vi "Retrieve Full Scale.vi"(8 "error in":errorcluster, 10 "Model Data":string, 11 "Alicat Device in":refnum<class "Alicat Device.lvclass">) -> (0 "error out":errorcluster, 1 "Type":string, 2 "Full Scale":sgl, 3 "Alicat Device out":refnum<class "Alicat Device.lvclass">, 4 "ModelOut":string)   [LabVIEW 2014, in "Alicat Lib.lvlib" / "Alicat Device.lvclass"]
doc: "The full scale of the device defines the input command for the setpoint (if the device is a controller). The setpoint command will use the full scale (FS) such that \n\nVal = SP*64000/FS"
uses:
  Alicat Device.lvclass
  Configurable Device/Configurable Device.lvclass/Configurable Device.ctl
  Alicat Device.lvclass/Alicat Device.ctl
  Configurable Device/Accessors/Write Model.vi
  Configurable Device/Accessors/Write SN.vi
  <vilib>/NI/Tools/String/Tools_String.lvlib
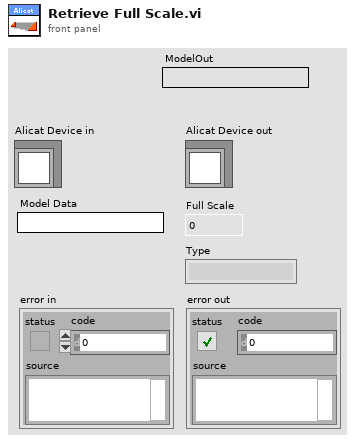
[diagram p1: front panel]
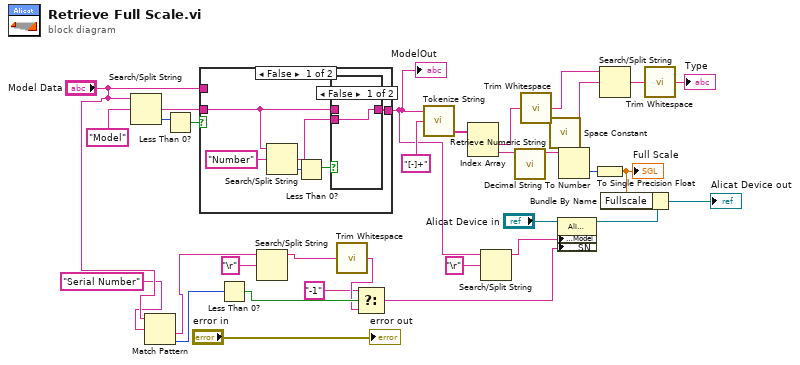
[diagram p0: block diagram]
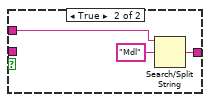
[diagram p3: hidden frame]
diagram:
  n1 = Search/Split String(string="Model Data", search string/char (-)="Model") -> (match + rest of string=w16:string, offset of match=w18:i32)  [unwired: 1 in, 1 out]
  n2 = Match Pattern(string="Model Data", regular expression="Serial Number" ("search string/char (-)")) -> (after substring=w10:string, offset past match=w9:i32)  [unwired: 1 in, 2 out]
  n3 = Less Than 0?(x=w18) -> (x < 0?=w17:bool)
  n4 = case shown="False" w17 {
    tunnel: "Model Data" -> [_ w43]
    tunnel: w16 -> [w35 _]
    tunnel: [w34 w41] -> w2
    frame False {
      n5 = Search/Split String(string=w35, search string/char (-)="Number") -> (match + rest of string=w33:string, offset of match=w37:i32)  [unwired: 1 in, 1 out]
      n6 = Less Than 0?(x=w37) -> (x < 0?=w36:bool)
      n7 = case shown="False" w36 {
        tunnel: w35 -> [_ w40]
        tunnel: [w39 w40] -> w34
        tunnel: w33 -> [w39 _]
        frame False {
        }
        frame True {
        }
      }
    }
    frame True {
      n8 = Search/Split String(string=w43, search string/char (-)="Mdl") -> (match + rest of string=w41:string)  [unwired: 1 in, 2 out]
    }
  }
  "ModelOut" <- w2
  n9 = Less Than 0?(x=w9) -> (x < 0?=w13:bool)
  n10 = Search/Split String(string=w10, search string/char (-)="\r") -> (substring before match=w7:string)  [unwired: 1 in, 2 out]
  n11 = call <vilib>:"Trim Whitespace.vi"("string"=w7) -> ("trimmed string"=w6:string)  [unwired: 1 in]
  n12 = Select(t="-1", s=w13, f=w6) -> (s? t:f=w4:string)
  n13 = call <vilib>:"Tokenize String.vi"("delimiter ([\\s\\t\\n\\r]+)"="[-]+" ("delimiter ([\\s\\t\\n\\r]+)"), "input string"=w2) -> ("token array"=w31:string[])  [unwired: 2 in, 1 out]
  n14 = Index Array(array=w31) -> (element #1=w27:string, element #2=w28:string)  [unwired: 2 in]
  n15 = Search/Split String(string=w2, search string/char (-)="\r") -> (substring before match=w1:string)  [unwired: 1 in, 2 out]
  n16 = call "Retrieve Numeric String.vi"("String in"=w28) -> ("Numeric String"=w30:string)  [unwired: 10 in]
  n17 = call <vilib>:"Trim Whitespace.vi"("string"=w27) -> ("trimmed string"=w26:string)  [unwired: 1 in]
  n18 = call <vilib>:"Space Constant.vi"() -> ("String"=w25:string)
  n19 = property class="Alicat Device"(reference="Alicat Device in", "Accessors:Model"=w1, "Accessors:SN"=w4) -> (reference out=w14:refnum<class "Alicat Device.lvclass">)  [unwired: 1 in, 1 out]
  n20 = Decimal String To Number(string=w30) -> (number=w29:i32)  [unwired: 2 in, 1 out]
  n21 = To Single Precision Float(number=w29) -> (single precision float=w22:sgl)
  "Full Scale" <- w22
  n22 = Search/Split String(string=w26, search string/char (-)=w25) -> (match + rest of string=w24:string)  [unwired: 1 in, 2 out]
  n23 = Bundle By Name(cluster=w14, "Fullscale"=w22) -> (→"Alicat Device out":refnum<class "Alicat Device.lvclass">)
  n24 = call <vilib>:"Trim Whitespace.vi"("string"=w24) -> ("trimmed string"=→"Type":string)  [unwired: 1 in]
  "error out" <- "error in"
